vi "App_Error Handle(FGV).vi"(6 "Error Handle Method(Enqueue)":T1=enum."Enqueue", 8 "error in":errorcluster) -> (0 "error out":errorcluster, 3 "Queue Ref.":refnum<queue>)   [LabVIEW 2015, in "Application 2.lvlib"]
uses:
  Application 2.lvlib
  Cloud Server/Data Def/Server_Error Handle Method.ctl
  Cloud Server/Cloud Server.lvlib
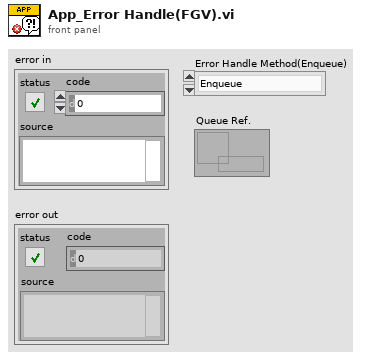
[diagram p1: front panel]
types:
  T1 = typedef "Cloud Server.lvlib/Server_Error Handle Method.ctl" = enum16{"Initialize", "Get Queue Ref.", "Enqueue", "Insert", "Flush", "Release"}
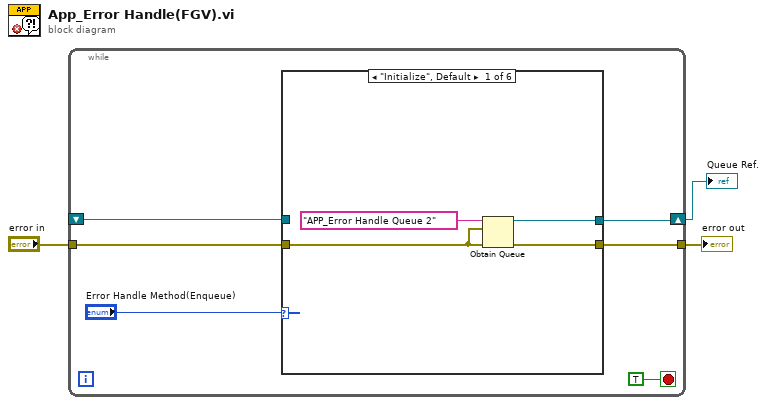
[diagram p0: block diagram]
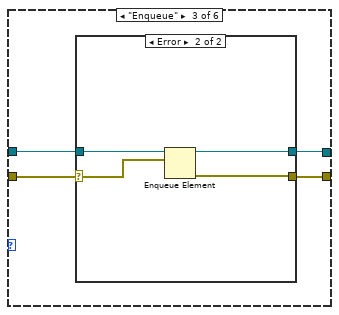
[diagram p3: hidden frame]
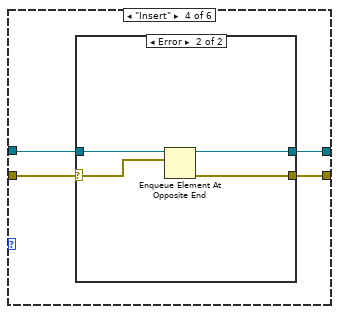
[diagram p5: hidden frame]
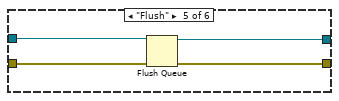
[diagram p7: hidden frame]
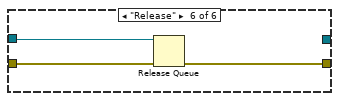
[diagram p8: hidden frame]
diagram:
  n1 = while {
    tunnel: "error in" -> [w8]
    tunnel: [w7] -> w2
    shift-right: [w6] -> w1
    shift-left: _ -> [w5]
    stop <- TRUE stop-if-true
    n2 = case shown="\"Initialize\", Default" "Error Handle Method(Enqueue)" {
      tunnel: w8 -> [w12 w14 w19 w27 w39 w42]
      tunnel: [w11 w14 w18 w29 w36 w40] -> w7
      tunnel: [w10 w15 w16 w28 w37 _] -> w6
      tunnel: w5 -> [_ w15 w17 w26 w38 w41]
      frame "Initialize", Default {
        n3 = Obtain Queue(name (unnamed)="APP_Error Handle Queue 2", element data type=w12, error in (no error)=w12) -> (queue out=w10:refnum<queue>, error out=w11:errorcluster)  [unwired: 2 in, 1 out]
      }
      frame "Get Queue Ref." {
      }
      frame "Enqueue" {
        n4 = case shown="Error" w19 {
          selector: w19 -> [w21 w22]
          tunnel: [w21 w25] -> w18
          tunnel: w17 -> [w20 w23]
          tunnel: [w20 w24] -> w16
          frame No Error {
          }
          frame Error {
            n5 = Enqueue Element(queue=w23, element=w22) -> (queue out=w24:refnum<queue>, error out=w25:errorcluster)  [unwired: 2 in, 1 out]
          }
        }
      }
      frame "Insert" {
        n6 = case shown="Error" w27 {
          selector: w27 -> [w31 w32]
          tunnel: [w31 w35] -> w29
          tunnel: w26 -> [w30 w33]
          tunnel: [w30 w34] -> w28
          frame No Error {
          }
          frame Error {
            n7 = Enqueue Element At Opposite End(queue=w33, element=w32) -> (queue out=w34:refnum<queue>, error out=w35:errorcluster)  [unwired: 2 in, 1 out]
          }
        }
      }
      frame "Flush" {
        n8 = Flush Queue(queue=w38, error in (no error)=w39) -> (queue out=w37:refnum<queue>, error out=w36:errorcluster)  [unwired: 1 out]
      }
      frame "Release" {
        n9 = Release Queue(queue=w41, error in (no error)=w42) -> (error out=w40:errorcluster)  [unwired: 1 in, 2 out]
      }
    }
  }
  "error out" <- w2
  "Queue Ref." <- w1
